vi "SL_Facade.vi"(0 "Data In":T5, 2 "Display State In":T3, 3 "Container State":T4) -> (6 "Data Out":T5, 7 "Display State Out":T3, 8 "Action":T2)   [LabVIEW 2019, in "SL_XControl.xctl"]
uses:
  SL_XControl.xctl
  SL_Data.ctl
  <vilib>/_xctls/Container State.ctl
  SL_State.ctl
  <vilib>/_xctls/Action.ctl
  <vilib>/_xctls/XControlSupport.lvlib
panel:
  out "Toggle":bool
  out "info":string
  in  "Refresh":bool
  in  "Login":bool
  in  "Edit":bool
  in  "Tag":T1
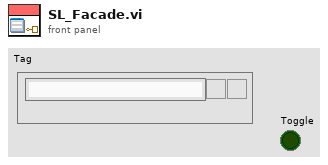
[diagram p1: front panel]
types:
  T1 = cluster{"Property":string, "Type":string, "Data":string}
  T2 = typedef "XControlSupport.lvlib/Action.ctl" = cluster{"Data Changed?":bool, "State Changed?":bool, "Action Name":string}
  T3 = typedef "SL_XControl.xctl/SL_State.ctl" = cluster{"Numeric":dbl}
  T4 = typedef "XControlSupport.lvlib/Container State.ctl" = cluster{"Indicator?":bool, "Run Mode?":bool, " Refnum":refnum<vi>}
  T5 = typedef "SL_XControl.xctl/SL_Data.ctl" = cluster{"Tag":string, "Type":string, "Data":string}
  T6 = enum8{"Enabled", "Disabled", "Disabled and Grayed Out"}
  T7 = cluster{"Name":string, "BaseURL":string, "AppKey":string, "Headers":string[], "Timeout":i32}
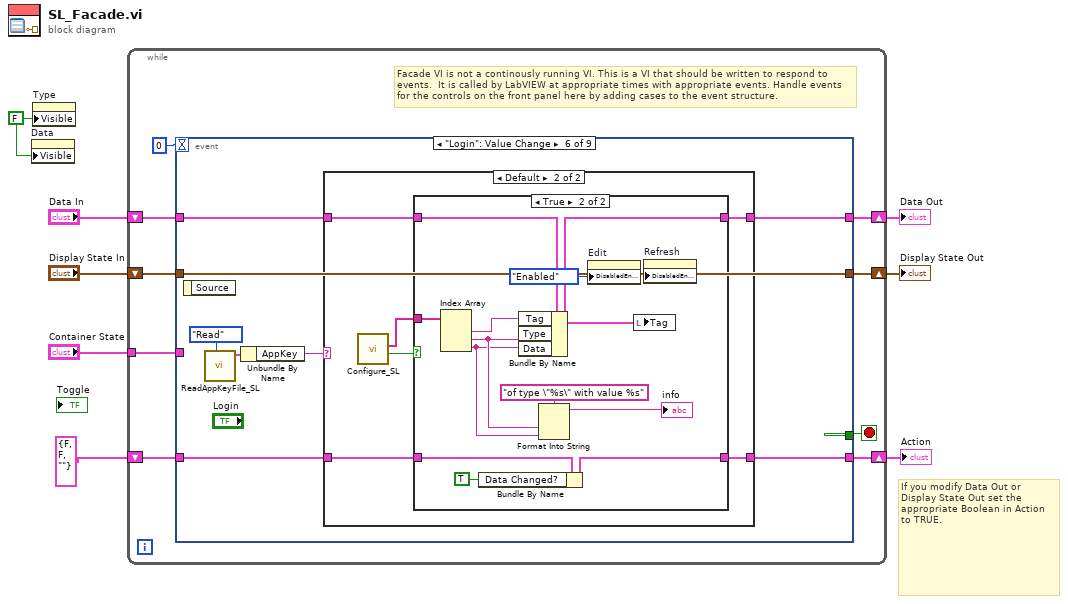
[diagram p0: block diagram]
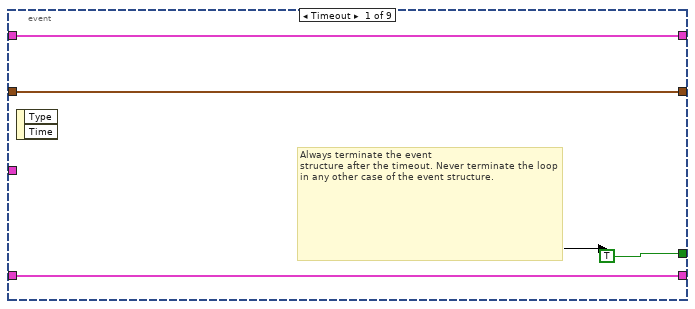
[diagram p2: hidden frame]
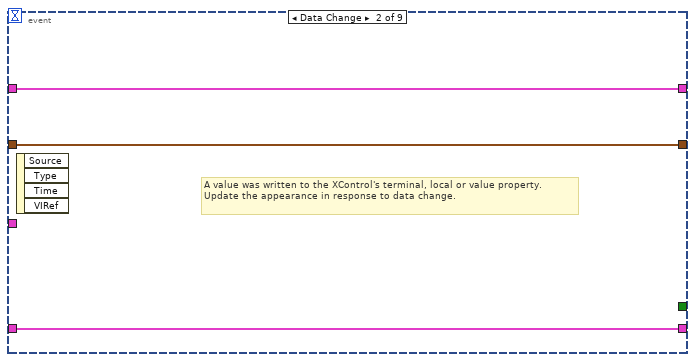
[diagram p3: hidden frame]
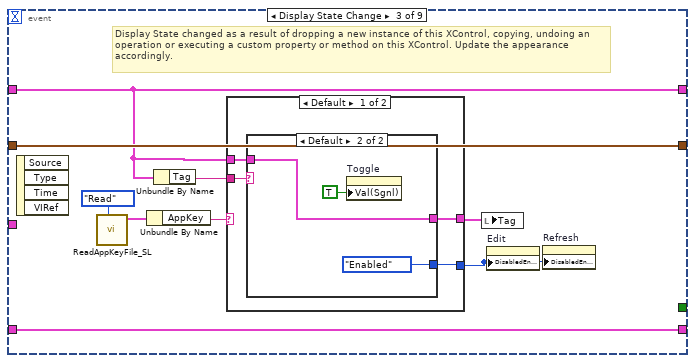
[diagram p4: hidden frame]
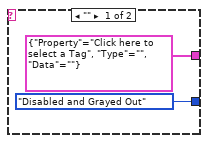
[diagram p5: hidden frame]
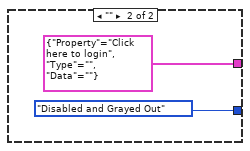
[diagram p6: hidden frame]
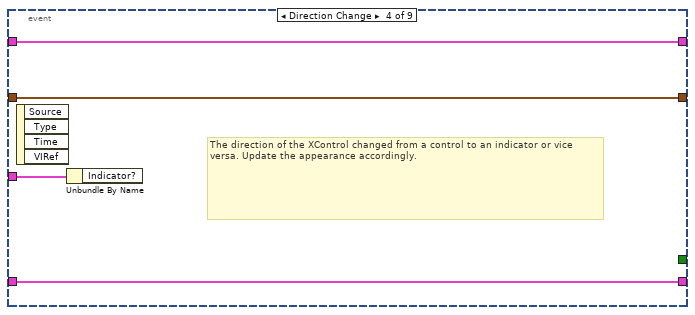
[diagram p7: hidden frame]
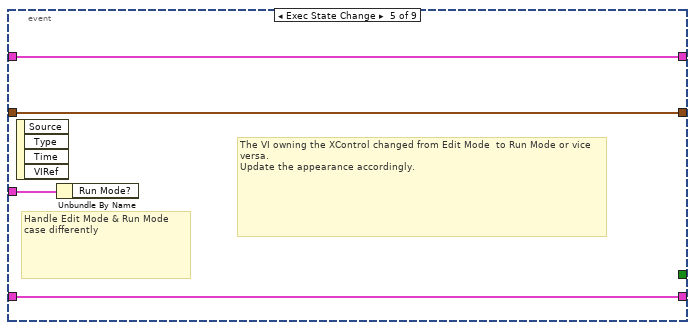
[diagram p8: hidden frame]
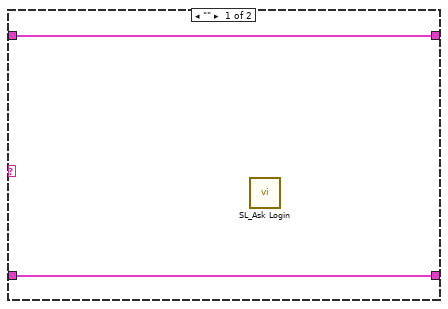
[diagram p9: hidden frame]
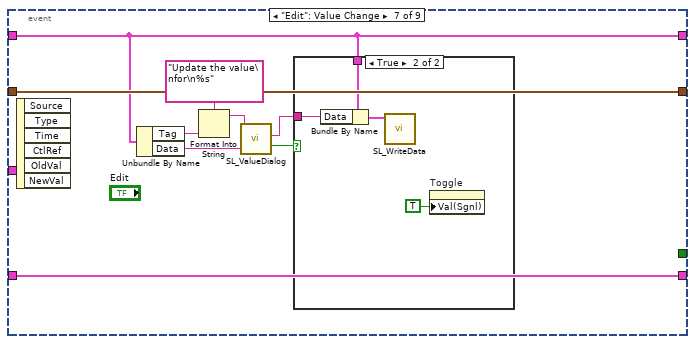
[diagram p11: hidden frame]
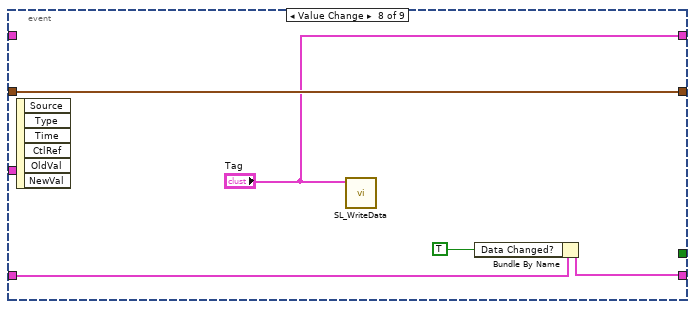
[diagram p13: hidden frame]
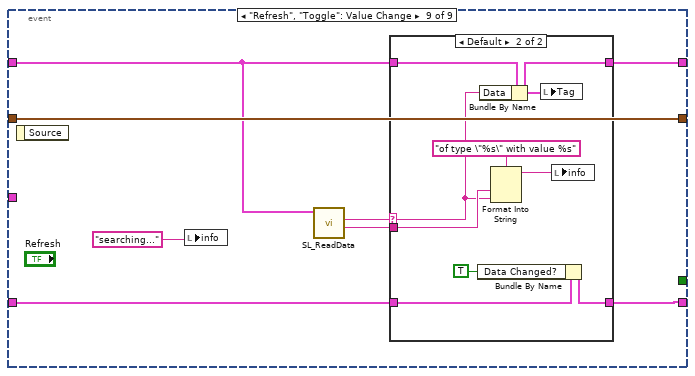
[diagram p14: hidden frame]
diagram:
  w1 = FALSE ("Visible")
  # "If you modify Data Out or\nDisplay State Out set the\nappropriate Boolean in Action\nto TRUE."
  n1 = property on="Data" class="Str"("Visible"=w1) -> ()  [unwired: 2 in, 2 out]
  n2 = property on="Type" class="Str"("Visible"=w1) -> ()  [unwired: 2 in, 2 out]
  n3 = while {
    shift-right: [w16] -> w5
    shift-left: "Display State In" -> [w17]
    tunnel: "Container State" -> [w13]
    shift-right: [w11] -> w8
    shift-left: "Data In" -> [w12]
    shift-right: [w9] -> w3
    shift-left: T2 {"Data Changed?"=FALSE, "State Changed?"=FALSE, "Action Name"=""} ("Action") -> [w10]
    stop <- w15 stop-if-true
    # "Facade VI is not a continously running VI. This is a VI that should be written to respond to events.  It is called by LabVIEW at appropriate times with appropriate events. Handle events for the controls on the front panel here by adding cases to the event structure."
    n4 = event shown="[5] \"Login\": Value Change" {
      selector: _ -> [_ _ _ _ _ _ _ _ _]
      dyn-events: _ -> [_ _ _ _ _ _ _ _ _]
      timeout: 0 -> [_ _ _ _ _ _ _ _ _]
      tunnel: w17 -> [w19 w23 w33 w47 w51 w60 w91 w100 w108]
      tunnel: [w19 w23 w33 w47 w51 w60 w91 w100 w108] -> w16
      tunnel: [TRUE _ _ _ _ _ _ _ _] -> w15
      tunnel: w13 -> [_ _ _ w48 w52 _ _ _ _]
      tunnel: w12 -> [w18 w24 w25 w46 w50 w57 w87 _ w104]
      tunnel: [w18 w24 w25 w46 w50 w56 w87 "Tag" w107] -> w11
      tunnel: [w20 w22 w32 w45 w49 w58 w90 w97 w105] -> w9
      tunnel: w10 -> [w20 w22 w32 w45 w49 w59 w90 w98 w106]
      event Timeout {
        # "Always terminate the event\nstructure after the timeout. Never terminate the loop in any other case of the event structure."
        n5 = event-data() -> ()  [unwired: 1 in, 2 out]
      }
      event Data Change {
        # "A value was written to the XControl's terminal, local or value property.\nUpdate the appearance in response to data change."
        n6 = event-data() -> ()  [unwired: 1 in, 4 out]
      }
      event Display State Change {
        # "Display State changed as a result of dropping a new instance of this XControl, copying, undoing an operation or executing a custom property or method on this XControl. Update the appearance accordingly."
        n7 = event-data() -> ()  [unwired: 1 in, 4 out]
        n8 = call "ReadAppKeyFile_SL.vi"("Task"=enum16{"Read", "Write"}."Read") -> ("Device Out"=w31:T7)  [unwired: 8 in, 2 out]
        n9 = Unbundle By Name(w31) -> ("AppKey"=w30:string)
        n10 = Unbundle By Name(w25) -> ("Tag"=w26:string)
        n11 = case shown="Default" w30 {
          tunnel: [w37 T1 {"Property"="Click here to login", "Type"="", "Data"=""} ("Tag")] -> w29
          tunnel: [w36 T6."Disabled and Grayed Out" ("Disabled")] -> w28
          tunnel: w26 -> [w35 _]
          tunnel: w25 -> [w34 _]
          frame Default {
            n12 = case shown="Default" w35 {
              tunnel: [T1 {"Property"="Click here to select a Tag", "Type"="", "Data"=""} ("Tag") w41] -> w37
              tunnel: [T6."Disabled and Grayed Out" ("Disabled") T6."Enabled" ("Disabled")] -> w36
              tunnel: w34 -> [_ w41]
              frame "" {
              }
              frame Default {
                n13 = property on="Toggle" class="Bool (strict)"("Val(Sgnl)"=TRUE ("Value (Signaling)")) -> ()  [unwired: 2 in, 2 out]
              }
            }
          }
          frame "" {
          }
        }
        n14 = local write "Tag"(w29) -> ()
        n15 = property on="Edit" class="Bool"("DisabledEnum"=w28) -> ()  [unwired: 2 in, 2 out]
        n16 = property on="Refresh" class="Bool"("DisabledEnum"=w28) -> ()  [unwired: 2 in, 2 out]
      }
      event Direction Change {
        # "The direction of the XControl changed from a control to an indicator or vice versa. Update the appearance accordingly."
        n17 = event-data() -> ()  [unwired: 1 in, 4 out]
        n18 = Unbundle By Name(w48) -> ()  [unwired: 1 out]
      }
      event Exec State Change {
        # "The VI owning the XControl changed from Edit Mode  to Run Mode or vice versa.\nUpdate the appearance accordingly."
        # "Handle Edit Mode & Run Mode\ncase differently"
        n19 = event-data() -> ()  [unwired: 1 in, 4 out]
        n20 = Unbundle By Name(w52) -> ()  [unwired: 1 out]
      }
      event "Login": Value Change {
        n21 = event-data() -> ()  [unwired: 1 in, 1 out]
        n22 = call "ReadAppKeyFile_SL.vi"("Task"=enum16{"Read", "Write"}."Read") -> ("Device Out"=w55:T7)  [unwired: 8 in, 2 out]
        n23 = Unbundle By Name(w55) -> ("AppKey"=w53:string)
        n24 = case shown="Default" w53 {
          tunnel: w59 -> [w61 w68]
          tunnel: [w61 w67] -> w58
          tunnel: w57 -> [w62 w66]
          tunnel: [w62 w65] -> w56
          frame "" {
            n25 = call "SL_Ask Login.vi"() -> ()  [unwired: 10 in, 2 out]
          }
          frame Default {
            n26 = call "Configure_SL.vi"() -> ("changed?"=w64:bool, "Property"=w63:string[])  [unwired: 10 in]
            n27 = case shown="True" w64 {
              tunnel: w66 -> [w70 w82]
              tunnel: [w70 w77] -> w65
              tunnel: w63 -> [_ w81]
              tunnel: w68 -> [w69 w79]
              tunnel: [w69 w78] -> w67
              frame False {
              }
              frame True {
                w72 = T6."Enabled" ("Disabled")
                n28 = Index Array(array=w81) -> (element #1=w71:string, element #2=w75:string, element #3=w74:string)  [unwired: 3 in]
                n29 = Bundle By Name(cluster=w79, "Data Changed?"=TRUE) -> (w78:T2)
                n30 = Bundle By Name(cluster=w82, "Tag"=w71, "Type"=w75, "Data"=w74) -> (w77:T5)
                n31 = Format Into String(format string="of type \"%s\" with value %s", w75, w74) -> (resulting string=→"info":string)  [unwired: 2 in, 1 out]
                n32 = property on="Edit" class="Bool"("DisabledEnum"=w72) -> ()  [unwired: 2 in, 2 out]
                n33 = local write "Tag"(w77) -> ()
                n34 = property on="Refresh" class="Bool"("DisabledEnum"=w72) -> ()  [unwired: 2 in, 2 out]
              }
            }
          }
        }
      }
      event "Edit": Value Change {
        n35 = event-data() -> ()  [unwired: 1 in, 6 out]
        n36 = Unbundle By Name(w87) -> ("Tag"=w84:string, "Data"=w89:string)
        n37 = Format Into String(format string="Update the value\nfor\n%s", w84) -> (resulting string=w83:string)  [unwired: 2 in, 1 out]
        n38 = call "SL_ValueDialog.vi"("Value"=w89, "Title"=w83) -> ("replace?"=w88:bool, "Value out"=w86:string)  [unwired: 8 in]
        n39 = case shown="True" w88 {
          tunnel: w87 -> [_ w95]
          tunnel: w86 -> [_ w94]
          frame False {
          }
          frame True {
            n40 = Bundle By Name(cluster=w95, "Data"=w94) -> (w93:T5)
            n41 = call "SL_WriteData.vi"("Tag"=w93) -> ()  [unwired: 11 in]
            n42 = property on="Toggle" class="Bool (strict)"("Val(Sgnl)"=TRUE ("Value (Signaling)")) -> ()  [unwired: 2 in, 2 out]
          }
        }
      }
      event "Tag.Data": Value Change {
        n43 = event-data() -> ()  [unwired: 1 in, 6 out]
        n44 = call "SL_WriteData.vi"("Tag"="Tag") -> ()  [unwired: 11 in]
        n45 = Bundle By Name(cluster=w98, "Data Changed?"=TRUE) -> (w97:T2)
      }
      event "Refresh", "Toggle": Value Change {
        n46 = event-data() -> ()  [unwired: 1 in, 1 out]
        n47 = local write "info"("searching..." ("info")) -> ()
        n48 = call "SL_ReadData.vi"("Tag"=w104) -> ("type"=w102:string, "value"=w103:string)  [unwired: 9 in]
        n49 = case shown="Default" w103 {
          selector: w103 -> [_ w113]
          tunnel: w104 -> [w110 w119]
          tunnel: [w110 w115] -> w107
          tunnel: w106 -> [w109 w118]
          tunnel: [w109 w117] -> w105
          tunnel: w102 -> [_ w114]
          frame "" {
          }
          frame Default {
            n50 = Bundle By Name(cluster=w118, "Data Changed?"=TRUE) -> (w117:T2)
            n51 = Bundle By Name(cluster=w119, "Data"=w113) -> (w115:T5)
            n52 = Format Into String(format string="of type \"%s\" with value %s", w114, w113) -> (resulting string=w111:string)  [unwired: 2 in, 1 out]
            n53 = local write "Tag"(w115) -> ()
            n54 = local write "info"(w111) -> ()
          }
        }
      }
    }
  }
  "Display State Out" <- w5
  "Data Out" <- w8
  "Action" <- w3
